vi "zurich_Lock_in_Messgearet.vi"(1 "refnum":refnum<file>, 2 "Numerisch":i8 min=0 max=2 step=1) -> ()   [LabVIEW 2019]
uses:
  Global/Global Variables/Data_Display_global.vi
  Instrument_Setup.vi
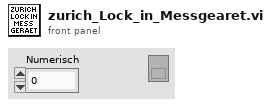
[diagram p1: front panel]
types:
  T1 = cluster{"Adress":string, "Load Settings from File":bool, "Output_Demod1":enum16{"Aux 1", "Aux 2", "Aux 3", "Aux 4"}, "Input_Demod1":enum16{"Sig In 1", "Curr In 1", "Trigger 1", "Trigger 2", "Aux Out 1", "Aux Out 2", "Aux Out 3", "Aux Out 4", "Aux In 1", "Aux In 2", "Constant"}, "Input_Mode_Demod1":enum16{"single ended", "differential"}, "Bandwith_Mode_Demod1":enum16{"TC", "BW NEP", "BW 3dB"}, "Bandw_Value_demod1":dbl, "Demod1_Range":dbl, "Demod1_Harmonic":dbl, "Trigger_Demod1":enum16{"Manual", "External"}, "osc1_freq":dbl, "osc1_amp":dbl, "Demod1_scaling":dbl, "osc2_freq":dbl, "osc2_amp":dbl, "osc3_freq":dbl, "osc3_amp":dbl, "osc4_freq":dbl, "osc4_amp":dbl, "Demod1_Phase (deg)":dbl, "Demod1_order":ext, "Demod1_coupling":enum16{"DC", "AC"}, "Demod1_shields":enum16{"Ground", "Float"}, "Demod1_input_resistance":enum16{"10M", "50"}, "Demod1_Ref_oscillator":ext, "Demod1_output_imp":enum16{"Disable", "Enable"}, "Demod1_output_diff":enum16{"Disable", "Enable"}, "Demod1_rate":dbl, "Demod1_Output_range":dbl, "Output_Demod2":enum16{"Aux 1", "Aux 2", "Aux 3", "Aux 4"}, "Demod2_input":enum16{"Sig In 1", "Curr In 1", "Trigger 1", "Trigger 2", "Aux Out 1", "Aux Out 2", "Aux Out 3", "Aux Out 4", "Aux In 1", "Aux In 2", "Constant"}, "Input_Mode_Demod2":enum16{"single ended", "differential"}, "Bandwith_Mode_Demod2":enum16{"TC", "BW NEP", "BW 3dB"}, "Bandw_Value_demod2":dbl, "Demod2_Range":dbl, "Demod2_Harmonic":dbl, "Trigger_Demod2":enum16{"Manual", "External"}, "Demod2_scaling":dbl, "Demod2_Phase (deg)":dbl, "Demod2_order":ext, "Demod2_coupling":enum16{"DC", "AC"}, "Demod2_shields":enum16{"Ground", "Float"}, "Demod2_input_resistance":enum16{"10M", "50"}, "Demod2_Ref_oscillator":ext, "Demod2_output_imp":enum16{"Disable", "Enable"}, "Demod2_output_diff":enum16{"Disable", "Enable"}, "Demod2_rate":dbl, "Demod2_Output_range":dbl, "Output_Demod3":enum16{"Aux 1", "Aux 2", "Aux 3", "Aux 4"}, "Demod3_input":enum16{"Sig In 1", "Curr In 1", "Trigger 1", "Trigger 2", "Aux Out 1", "Aux Out 2", "Aux Out 3", "Aux Out 4", "Aux In 1", "Aux In 2", "Constant"}, "Input_Mode_Demod3":enum16{"single ended", "differential"}, "Bandwith_Mode_Demod2":enum16{"TC", "BW NEP", "BW 3dB"}, "Bandw_Value_demod3":dbl, "Demod3_Range":dbl, "Demod3_Harmonic":dbl, "Trigger_Demod3":enum16{"Manual", "External"}, "Demod3_scaling":dbl, "Demod3_Phase (deg)":dbl, "Demod3_order":ext, "Demod3_coupling":enum16{"DC", "AC"}, "Demod3_shields":enum16{"Ground", "Float"}, "Demod3_input_resistance":enum16{"10M", "50"}, "Demod3_Ref_oscillator":ext, "Demod3_output_imp":enum16{"Disable", "Enable"}, "Demod3_output_diff":enum16{"Disable", "Enable"}, "Demod3_rate":dbl, "Demod3_Output_range":dbl, "Output_Demod4":enum16{"Aux 1", "Aux 2", "Aux 3", "Aux 4"}, "Demod4_input":enum16{"Sig In 1", "Curr In 1", "Trigger 1", "Trigger 2", "Aux Out 1", "Aux Out 2", "Aux Out 3", "Aux Out 4", "Aux In 1", "Aux In 2", "Constant"}, "Input_Mode_Demod4":enum16{"single ended", "differential"}, "Bandwith_Mode_Demod4":enum16{"TC", "BW NEP", "BW 3dB"}, "Bandw_Value_demod4":dbl, "Demod4_Range":dbl, "Demod4_Harmonic":dbl, "Trigger_Demod4":enum16{"Manual", "External"}, "Demod4_scaling":dbl, "Demod4_Phase (deg)":dbl, "Demod4_order":ext, "Demod4_coupling":enum16{"DC", "AC"}, "Demod4_shields":enum16{"Ground", "Float"}, "Demod4_input_resistance":enum16{"10M", "50"}, "Demod4_Ref_oscillator":ext, "Demod4_output_imp":enum16{"Disable", "Enable"}, "Demod4_output_diff":enum16{"Disable", "Enable"}, "Demod4_rate":dbl, "Demod4_Output_range":dbl, "Oscillator1_Amp_units":enum16{"Vpk", "Vrms", "VdBm"}, "Oscillator4_Amp_units":enum16{"Vpk", "Vrms", "VdBm"}, "Oscillator2_Amp_units":enum16{"Vpk", "Vrms", "VdBm"}, "Oscillator3_Amp_units":enum16{"Vpk", "Vrms", "VdBm"}, "Demod1_sync_filter":enum16{"Disable", "Enable"}, "Demod 1 (on/off)":bool, "Demod 2 (on/off) ":bool, "Demod 3 (on/off) ":bool, "Demod 4 (on/off) ":bool, " Sigouts 1 (on/off)":bool, " Sigouts 2 (on/off) ":bool, " Sigouts 3 (on/off)":bool, " Sigouts 4 (on/off) ":bool, "Demod2_sync_filter":enum16{"Disable", "Enable"}, "Demod1_auto_outp_rang":enum16{"Disable", "Enable"}, "Demod2_auto_outp_rang ":enum16{"Disable", "Enable"}}
  T2 = typedef "zurichinstMonitor.ctl" = cluster{"Dmod 1 X":dbl, "Dmod 1 Y":dbl, "Dmod 1 R":dbl, "Dmod 1 Theta":dbl, "Update Oscillators":bool, "Dmod 2 X":dbl, "Dmod 2 R":dbl, "Dmod 2 Y":dbl, "Dmod 2 Theta":dbl}
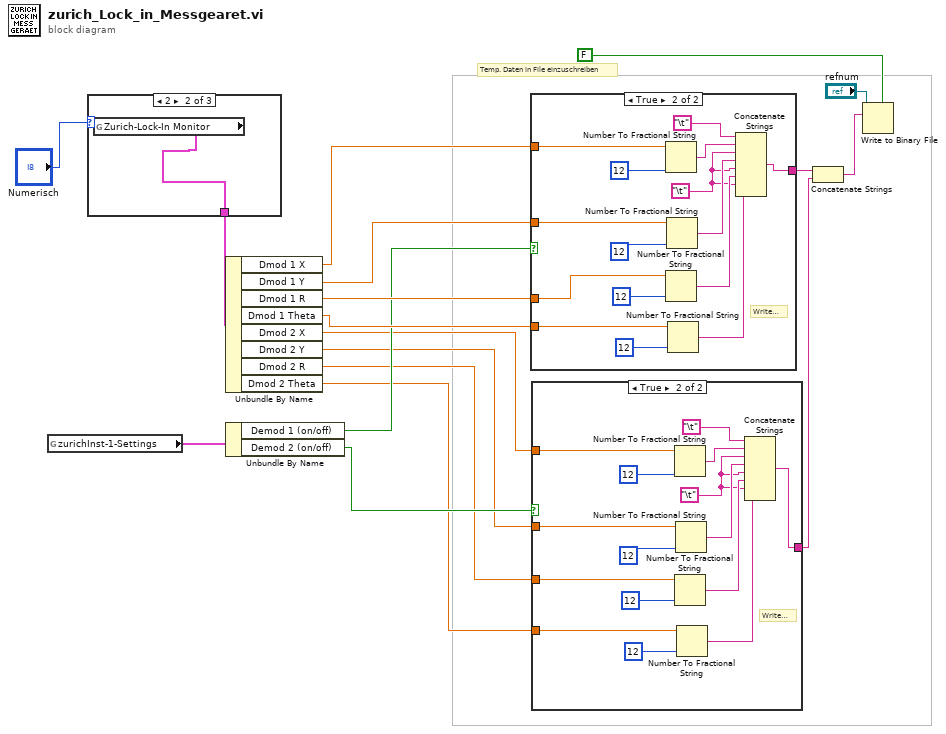
[diagram p0: block diagram]
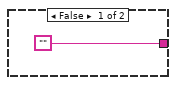
[diagram p2: hidden frame]
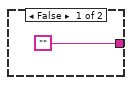
[diagram p3: hidden frame]
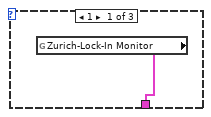
[diagram p4: hidden frame]
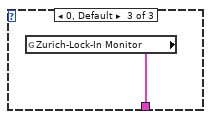
[diagram p5: hidden frame]
diagram:
  # "Temp. Daten in File einzuschreiben"
  n1 = global read "Instrument_Setup.vi" "zurichInst-1-Settings"() -> (w8:T1)
  n2 = case shown="2" "Numerisch" {
    tunnel: [w19 w20 w21] -> w15
    frame 1 {
      n3 = global read "Data_Display_global.vi" "Zurich-Lock-In Monitor"() -> (w19:T2)
    }
    frame 2 {
      n4 = global read "Data_Display_global.vi" "Zurich-Lock-In Monitor"() -> (w20:T2)
    }
    frame 0, Default {
      n5 = global read "Data_Display_global.vi" "Zurich-Lock-In Monitor"() -> (w21:T2)
    }
  }
  n6 = Unbundle By Name(w15) -> ("Dmod 1 X"=w13:dbl, "Dmod 1 Y"=w14:dbl, "Dmod 1 R"=w12:dbl, "Dmod 1 Theta"=w11:dbl, "Dmod 2 X"=w5:dbl, "Dmod 2 Y"=w4:dbl, "Dmod 2 R"=w3:dbl, "Dmod 2 Theta"=w2:dbl)
  n7 = Unbundle By Name(w8) -> ("Demod 1 (on/off)"=w7:bool, "Demod 2 (on/off)"=w6:bool)
  n8 = case shown="True" w7 {
    tunnel: w14 -> [_ w32]
    tunnel: w13 -> [_ w31]
    tunnel: w12 -> [_ w28]
    tunnel: w11 -> [_ w27]
    tunnel: ["" w23] -> w9
    frame False {
    }
    frame True {
      w25 = "\t"
      # "Write File"
      n9 = Number To Fractional String(number=w31, precision (6)=i16 12) -> (F-format string=w36:string)  [unwired: 2 in]
      n10 = Number To Fractional String(number=w28, precision (6)=i16 12) -> (F-format string=w26:string)  [unwired: 2 in]
      n11 = Number To Fractional String(number=w32, precision (6)=i16 12) -> (F-format string=w35:string)  [unwired: 2 in]
      n12 = Number To Fractional String(number=w27, precision (6)=i16 12) -> (F-format string=w24:string)  [unwired: 2 in]
      n13 = Concatenate Strings("\t", w36, w25, w35, w25, w26, w25, w24) -> (w23:string)
    }
  }
  n14 = case shown="True" w6 {
    tunnel: w5 -> [_ w43]
    tunnel: w4 -> [_ w42]
    tunnel: w3 -> [_ w41]
    tunnel: w2 -> [_ w40]
    tunnel: ["" w39] -> w1
    frame False {
    }
    frame True {
      w45 = "\t"
      # "Write File"
      n15 = Number To Fractional String(number=w43, precision (6)=i16 12) -> (F-format string=w52:string)  [unwired: 2 in]
      n16 = Number To Fractional String(number=w41, precision (6)=i16 12) -> (F-format string=w46:string)  [unwired: 2 in]
      n17 = Number To Fractional String(number=w42, precision (6)=i16 12) -> (F-format string=w51:string)  [unwired: 2 in]
      n18 = Number To Fractional String(number=w40, precision (6)=i16 12) -> (F-format string=w44:string)  [unwired: 2 in]
      n19 = Concatenate Strings("\t", w52, w45, w51, w45, w46, w45, w44) -> (w39:string)
    }
  }
  n20 = Concatenate Strings(w9, w1) -> (w10:string)
  n21 = Write to Binary File ("Write File")(file (use dialog)="refnum", data=w10, 5:FALSE ("prepend array or string size? (T)")) -> ()  [unwired: 3 in, 3 out]
